vi "Mark Unmark Source Only.vi"() -> ()   [LabVIEW 2014]
uses:
  <vilib>/Utility/error.llb/DialogType.ctl
panel:
  in  "done2":bool
  out "Progress 2":dbl(slide) scale=0.0..1.0
  in  "Abort":bool
  in  "Done":bool
  in  "Run":bool
  out "Status":string
  in  "Set Separate Compiled Code":bool=TRUE
  in  "VI, Library, LLB, Folder or File List Path":path=path "C:/dev/sourceonlydist/vi.lib"
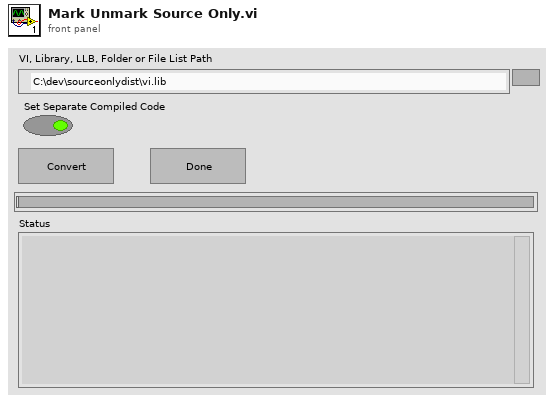
[diagram p1: front panel]
types:
  T1 = enum8{"Enabled", "Disabled", "Disabled and Grayed Out"}
  T2 = typedef "Librarian File Info Out.ctl" = cluster{"creation date":u32, "last mod date":u32, "type":string, "creator":string, "LV version":i32, "size":i32, "top level":bool}
  T3 = typedef "DialogType.ctl" = u16
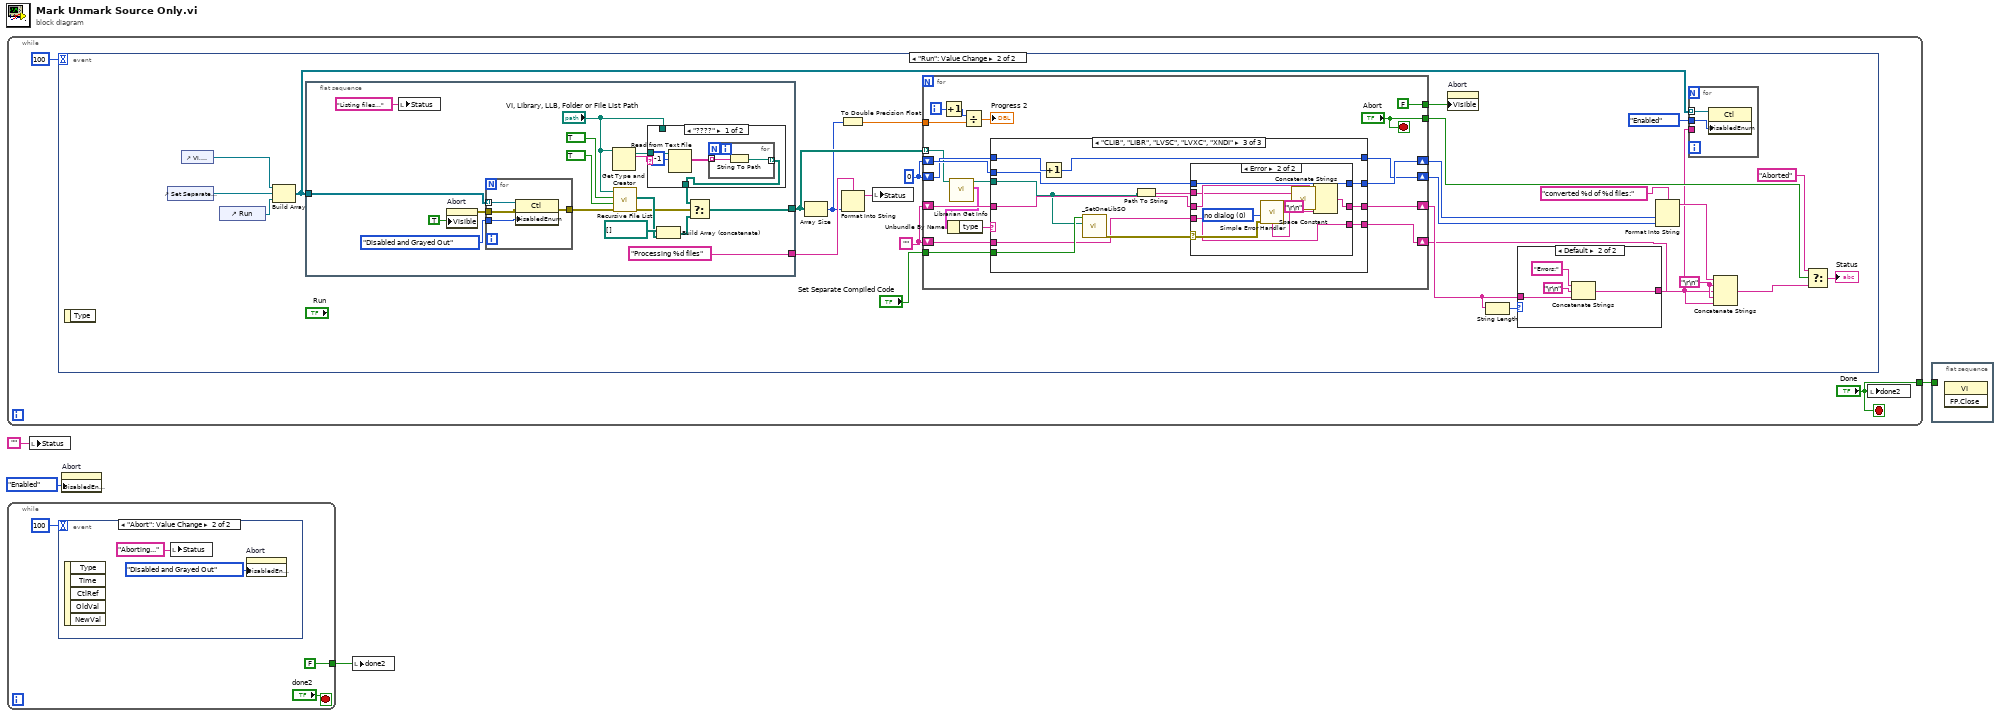
[diagram p0: block diagram]
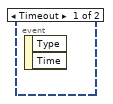
[diagram p2: hidden frame]
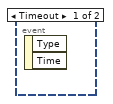
[diagram p3: hidden frame]
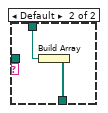
[diagram p4: hidden frame]
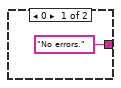
[diagram p5: hidden frame]
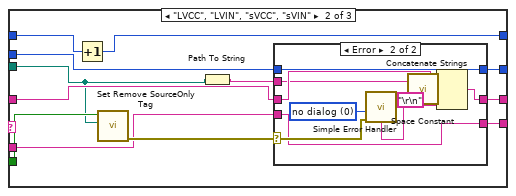
[diagram p7: hidden frame]
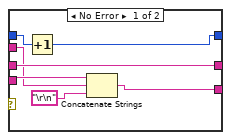
[diagram p8: hidden frame]
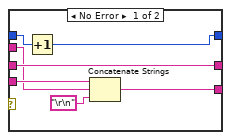
[diagram p9: hidden frame]
diagram:
  n1 = while {
    tunnel: ["Done"] -> w4
    stop <- "Done" stop-if-true
    n2 = event shown="[1] \"Run\": Value Change" {
      selector: _ -> [_ _]
      dyn-events: _ -> [_ _]
      timeout: 100 -> [_ _]
      event Timeout {
        n3 = event-data() -> ()  [unwired: 1 in, 2 out]
      }
      event "Run": Value Change {
        w8 = "\r\n"
        w10 = ""
        w27 = 0
        n4 = event-data() -> ()  [unwired: 1 in, 1 out]
        n5 = control-ref of="Set Separate Compiled Code"() -> (w19:refnum<vi>)
        n6 = control-ref of="VI, Library, LLB, Folder or File List Path"() -> (w18:refnum<vi>)
        n7 = control-ref of="Run"() -> (w20:refnum<vi>)
        n8 = Build Array(w18, w19, w20) -> (w17:refnum<vi>[])
        n9 = flat-sequence {
          tunnel: [w47] -> w25
          tunnel: ["Processing %d files"] -> w22
          tunnel: w17 -> [w44]
          frame #0 {
            n10 = local write "Status"("Listing files..." ("Status")) -> ()
            n11 = property on="Abort" class="Bool"("Visible"=TRUE) -> (error out=w42:errorcluster)  [unwired: 2 in, 1 out]
            n12 = for {
              tunnel: w44 -> [w65] mode=indexing
              tunnel: T1."Disabled and Grayed Out" ("Disabled") -> [w64]
              tunnel: w42 -> [w63]
              tunnel: [w62] -> w41
              n13 = property on="Property Node" class="Ctl"(reference=w65, error in=w63, "DisabledEnum"=w64) -> (error out=w62:errorcluster)  [unwired: 1 out]
            }
            n14 = Get Type and Creator(7:"VI, Library, LLB, Folder or File List Path") -> (2:w39:string, 3:w37:path)  [unwired: 1 in, 2 out]
            n15 = call <vilib>:"Recursive File List.vi"("error in (no error)"=w41, "Continue Recursing on Error? (F)"=TRUE, "Treat LLBs as Folders?"=TRUE, "Folder Path"="VI, Library, LLB, Folder or File List Path") -> ("error out"=w40:errorcluster, "All Files in Dir"=w50:path[])  [unwired: 3 in, 3 out]
            n16 = case shown="\"????\"" w39 {
              tunnel: "VI, Library, LLB, Folder or File List Path" -> [_ w61]
              tunnel: w37 -> [w57 _]
              tunnel: [w54 w60] -> w36
              frame "????" {
                n17 = Read from Text File(file (use dialog)=w57, count=-1) -> (text=w55:string[])  [unwired: 2 in, 3 out]
                n18 = for {
                  tunnel: w55 -> [w59] mode=indexing
                  tunnel: [w58] -> w54 mode=indexing
                  n19 = String To Path(string=w59) -> (path=w58:path)
                }
              }
              frame Default {
                n20 = Build Array(w61) -> (w60:path[])
              }
            }
            n21 = Build Array (concatenate)(path[] [] ("All Files in Dir"), w50) -> (w49:path[])
            n22 = Select(t=w36, s=w40, f=w49) -> (s? t:f=w47:path[])
          }
        }
        n23 = Array Size(array=w25) -> (size(s)=w21:i32)
        n24 = To Double Precision Float(number=w21) -> (double precision float=w24:dbl)
        n25 = Format Into String(format string=w22, w21) -> (resulting string=w23:string)  [unwired: 2 in, 1 out]
        n26 = local write "Status"(w23) -> ()
        n27 = for {
          tunnel: w25 -> [w74] mode=indexing
          shift-right: [w88] -> w32
          shift-left: w27 -> [w89]
          shift-right: [w86] -> w31
          shift-left: w27 -> [w87]
          shift-right: [w84] -> w29
          shift-left: w10 -> [w85]
          tunnel: [FALSE ("Visible")] -> w26
          tunnel: w24 -> [w81]
          tunnel: ["Abort"] -> w15
          tunnel: "Set Separate Compiled Code" -> [w79]
          shift-right: [w77] -> w7
          shift-left: w10 -> [w78]
          i -> [w76]
          stop <- "Abort" stop-if-true
          n28 = Increment(x=w76) -> (x+1=w75:i32)
          n29 = call <vilib>:"Librarian Get Info.vi"("path"=w74) -> ("file information"=w72:T2, "dup path"=w73:path)  [unwired: 8 in, 1 out]
          n30 = Unbundle By Name(w72) -> ("type"=w71:string)
          n31 = Divide(x=w75, y=w81) -> (x/y=→"Progress 2":dbl)
          n32 = case shown="\"CLIB\", \"LIBR\", \"LVSC\", \"LVXC\", \"XNDI\"" w71 {
            tunnel: w89 -> [w92 w104 w133]
            tunnel: [w92 w103 w132] -> w88
            tunnel: w73 -> [_ w97 w125]
            tunnel: w87 -> [w93 w102 w131]
            tunnel: [w93 w101 w130] -> w86
            tunnel: w85 -> [w91 w99 w128]
            tunnel: [w91 w100 w129] -> w84
            tunnel: w79 -> [_ w98 w127]
            tunnel: w78 -> [w90 w95 w124]
            tunnel: [w90 w94 w123] -> w77
            frame Default {
            }
            frame "LVCC", "LVIN", "sVCC", "sVIN" {
              n33 = Increment(x=w102) -> (x+1=w101:i32)
              n34 = call <vilib>:"Set Remove SourceOnly Tag.vi"("VI Path"=w97, "Set"=w98) -> ("error out"=w105:errorcluster)  [unwired: 9 in]
              n35 = Path To String(path=w97) -> (string=w96:string)
              n36 = case shown="Error" w105 {
                selector: w105 -> [_ w120]
                tunnel: w104 -> [w112 w122]
                tunnel: [w111 w122] -> w103
                tunnel: [w110 w117] -> w100
                tunnel: w99 -> [w110 w115]
                tunnel: w96 -> [w108 w114]
                tunnel: w95 -> [w109 w113]
                tunnel: [w106 w113] -> w94
                frame No Error {
                  n37 = Increment(x=w112) -> (x+1=w111:i32)
                  n38 = Concatenate Strings(w109, w108, "\r\n") -> (w106:string)
                }
                frame Error {
                  w121 = T3 0 items=["no dialog", "OK message", "continue or stop message", "OK message + warnings", "continue/stop + warnings"] ("type of dialog (OK msg:1)")
                  n39 = call <vilib>:"Simple Error Handler.vi"("type of dialog (OK msg:1)"=w121, "error in (no error)"=w120) -> ("message"=w119:string)  [unwired: 3 in, 4 out]
                  n40 = call <vilib>:"Space Constant.vi"() -> ("String"=w116:string)
                  n41 = Concatenate Strings(w115, w114, w116, w119, "\r\n") -> (w117:string)
                }
              }
            }
            frame "CLIB", "LIBR", "LVSC", "LVXC", "XNDI" {
              n42 = Increment(x=w131) -> (x+1=w130:i32)
              n43 = call "_SetOneLibSO.vi"("Path"=w125, "Set"=w127) -> ("error out"=w134:errorcluster)  [unwired: 7 in]
              n44 = Path To String(path=w125) -> (string=w126:string)
              n45 = case shown="Error" w134 {
                selector: w134 -> [_ w149]
                tunnel: w133 -> [w141 w151]
                tunnel: [w140 w151] -> w132
                tunnel: [w139 w146] -> w129
                tunnel: w128 -> [w139 w144]
                tunnel: w126 -> [w137 w143]
                tunnel: w124 -> [w138 w142]
                tunnel: [w135 w142] -> w123
                frame No Error {
                  n46 = Increment(x=w141) -> (x+1=w140:i32)
                  n47 = Concatenate Strings(w138, w137, "\r\n") -> (w135:string)
                }
                frame Error {
                  w150 = T3 0 items=["no dialog", "OK message", "continue or stop message", "OK message + warnings", "continue/stop + warnings"] ("type of dialog (OK msg:1)")
                  n48 = call <vilib>:"Simple Error Handler.vi"("type of dialog (OK msg:1)"=w150, "error in (no error)"=w149) -> ("message"=w148:string)  [unwired: 3 in, 4 out]
                  n49 = call <vilib>:"Space Constant.vi"() -> ("String"=w145:string)
                  n50 = Concatenate Strings(w144, w143, w145, w148, "\r\n") -> (w146:string)
                }
              }
            }
          }
        }
        n51 = property on="Abort" class="Bool"("Visible"=w26) -> ()  [unwired: 2 in, 2 out]
        n52 = String Length(string=w29) -> (length=w30:i32)
        n53 = case shown="Default" w30 {
          tunnel: w29 -> [_ w68]
          tunnel: ["No errors." w67] -> w9
          frame 0 {
          }
          frame Default {
            n54 = Concatenate Strings("Errors:", "\r\n", w68) -> (w67:string)
          }
        }
        n55 = Format Into String(format string="converted %d of %d files:", w32, w31) -> (resulting string=w28:string)  [unwired: 2 in, 1 out]
        n56 = for {
          tunnel: w17 -> [w35] mode=indexing
          tunnel: T1."Enabled" ("Disabled") -> [w34]
          tunnel: w9 -> [_]
          n57 = property on="Property Node" class="Ctl"(reference=w35, "DisabledEnum"=w34) -> ()  [unwired: 1 in, 2 out]
        }
        n58 = Concatenate Strings(w28, w8, w7, w8, w9) -> (w13:string)
        n59 = Select(t="Aborted" ("format string"), s=w15, f=w13) -> (s? t:f=→"Status":string)
      }
    }
    n60 = local write "done2"("Done") -> ()
  }
  n61 = while {
    tunnel: [FALSE] -> w1
    stop <- "done2" stop-if-true
    n62 = event shown="[1] \"Abort\": Value Change" {
      selector: _ -> [_ _]
      dyn-events: _ -> [_ _]
      timeout: 100 -> [_ _]
      event Timeout {
        n63 = event-data() -> ()  [unwired: 1 in, 2 out]
      }
      event "Abort": Value Change {
        n64 = event-data() -> ()  [unwired: 1 in, 5 out]
        n65 = local write "Status"("Aborting..." ("Status")) -> ()
        n66 = property on="Abort" class="Bool"("DisabledEnum"=T1."Disabled and Grayed Out" ("Disabled")) -> ()  [unwired: 2 in, 2 out]
      }
    }
  }
  n67 = local write "Status"("") -> ()
  n68 = property on="Abort" class="Bool"("DisabledEnum"=T1."Enabled" ("Disabled")) -> ()  [unwired: 2 in, 2 out]
  n69 = local write "done2"(w1) -> ()
  n70 = flat-sequence {
    tunnel: w4 -> [_]
    frame #0 {
      n71 = invoke class="VI" method="FP.Close"() -> ()  [unwired: 3 in, 3 out]
    }
  }
